vi "insideBounds.vi"(8 "error in (no error)":errorcluster, 10 "Rectangle":T1, 11 "point":cluster{"X":dbl, "Y":dbl}) -> (0 "error out":errorcluster, 2 "inside":bool)   [LabVIEW 2010, in "OccupancyMap.lvclass"]
uses:
  OccupancyMap.lvclass
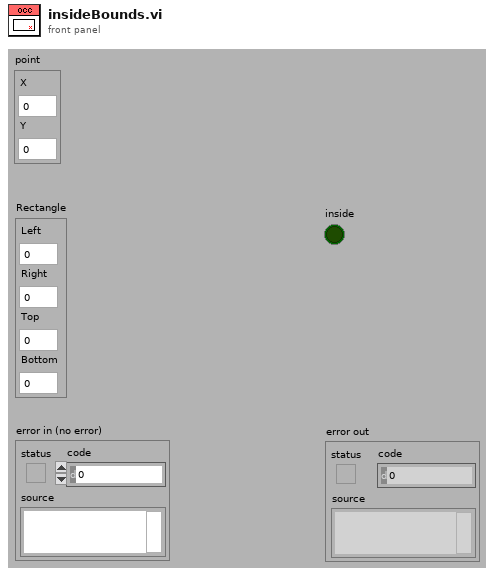
[diagram p1: front panel]
types:
  T1 = cluster{"Left":dbl, "Right":dbl, "Top":dbl, "Bottom":dbl}
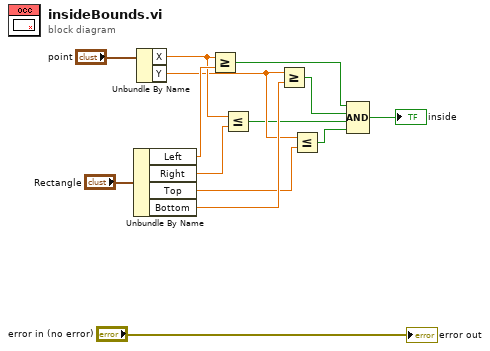
[diagram p0: block diagram]
diagram:
  n1 = Unbundle By Name("Rectangle") -> ("Left"=w12:dbl, "Right"=w11:dbl, "Top"=w7:dbl, "Bottom"=w9:dbl)
  n2 = Unbundle By Name("point") -> ("X"=w10:dbl, "Y"=w8:dbl)
  n3 = Greater Or Equal?(x=w10, y=w12) -> (x >= y?=w6:bool)
  n4 = Less Or Equal?(x=w10, y=w11) -> (x <= y?=w4:bool)
  n5 = Greater Or Equal?(x=w8, y=w9) -> (x >= y?=w5:bool)
  n6 = Less Or Equal?(x=w8, y=w7) -> (x <= y?=w3:bool)
  n7 = Compound Arithmetic op=AND(w6, w5, w4, w3) -> (→"inside":bool)
  "error out" <- "error in (no error)"
